vi "HEWH Solenoid Bank.vi"(0 "Test Fixture Hardware":T1={"Power "={"Yokogawa"={"WT210"={"Sample Rate (1: 0.25s)"=1, "A Range (12: 20A)"=11, "V Range (6: 600V)"=4, "Power VISA Yokogawa WT210"="WT210"}, "WT500"={"Power VISA Yokogawa WT500"="", "V Range (8: 1000V)"=6, "I Range (7: 40A)"=7, "Update Rate (3: 500ms)"=2}, "WT310_2"={"Sample Rate (1: 0.25s)"=1, "A Range (12: 20A)"=11, "V Range (6: 600V)"=4, "Power VISA Yokogawa WT310_2"="WT310_2"}, "WT310_3"={"Sample Rate (1: 0.25s)"=1, "A Range (12: 20A)"=11, "V Range (6: 600V)"=4, "Power VISA Yokogawa WT310_3"="WT310_3"}}, "Aplus"={"Aplus IP Address"="192.168.1.101", "Remote Port"=502, "Instrument"="APLUS", "Instr Driver Revision"="1.03.0053"}, "Power Limits"={"Crest Factor"={"Upper Limit"=1.49, "Lower Limit"=1.34}, "Harmonic Content"={"Uthd"=2.0}, "Voltage"={"% Error"=2.0}, "Stability"={"<1 Watt "={"Wattage"=1.0, "Slope (mW/H)"=10.0}, ">1 Watt"={"1%Power/Hour"=1.0}}}, "Nominal Voltage"=120, "Time Limit (s)"=10800.0, "Power Variation Limit (%)"=50.0, "Power Supply"={"Chroma 61605"="CHROMA", "Use Chroma?"=FALSE}}, "Weight Scale"={"Com Options"={"IND560Scale VISA"="IND560", "IP Address"="", "Remote Port"=502, "Setra Scale VISA"="SETRA", "GSE 350"="GSE350"}, "Select Scale"=""}, "Flow Rates"={"Laurel Cold IP Address"="", "Laurel Hot IP Address"="", "Hot Water Laurel VISA"="LaurelMeter_Hot", "Cold Water Laurel VISA"="LaurelMeter_Cold", "Remote Port"=0, "Laurel Communication Type"="", "Meters To Collect (Hot Cold)"="", "HOT Laurel Reference"=refnum, "COLD Laurel Reference"=refnum, "Modbus Hot Ref"=refnum}, "Analog Data"={"Agilent"={"Agilent 34972_1"="34972A_1", "Agilent 34972_2"="34972A_2", "Agilent 34972_3"="34972A_3", "Agilent 34972_4"="34972A_3", "Agilent 34972_5"="34972A_3", "Agilent 34972_6"="34972A_3", "Agilent Gain"=0.0, "TC Type (K,J,T)"="", "Instrument IDN?"="", "TC Channels-List"="", "Analog Channels-List"="", "Agilent Cluster Array"=[], "TC Channels-List 2"="", "Analog Channels-List 2"=""}, "Yokogawa"={"MW100"="MW100", "Intellifaucet"=FALSE}, "Select Analog"="", "TC Coefficients"={"TC Coefficients 1"=[], "TC Coefficients 2"=[], "TC Coefficients 3"=[], "TC Coefficients 4"=[], "TC Coefficients 5"=[], "TC Coefficients 6"=[], "TC Coefficients 7"=[]}, "NI Tasks (Dryer DOE)"=["TC Temps-Module 1", "TC Temps-Module 2", "TC Temps-Module 3", "TC Temps-Module 4", "TC Temps-Module 5", "Gas and Temp-Module 6", "AC_DC Events-Module 7"], "Laurel Analog"={"Laurel IP (Water Temp)"="", "Laurel IP (Pressure)"=""}}, "Viasala Temperature & Humidity"={"IP Address 1"="", "Remote Port"=0, "IP Address 2"="", "IP Address 3"="", "Viasala Modbus"=refnum, "Probe Number"=0}, "Gas Meter"={"Gas Meter 1"="COM3", "Gas Meter 2"="COM4", "Gas Meter 3"="COM5", "Gas Meter 4"="COM6", "Gas Meter 5"="COM7", "Gas Meter 6"="COM8", "Data Frame Format"={"Absolute Pressure"=FALSE, "Gauge/Diff. Pressure"=FALSE, "Barometric Pressure"=FALSE, "Temperature"=FALSE, "Volumetric"=FALSE, "Mass"=FALSE, "Setpoint"=FALSE, "Valve Drive"=FALSE, "Totalizer"=FALSE, "Totalizer Timer"=FALSE, "Totalizer Average Flow"=FALSE, "Totalizer Peak Flow"=FALSE, "Gas Selected"=FALSE, "Tot. Timer Format"=0}, "Measurement Units"={"Software Rev"="", "Model Number"="", "Manufacturer Info"="", "Software Sub-Rev"="", "Board Rev"="", "Units of Measure Input"={"Abs. Pressure"="", "Gauge/Diff. Press."="", "Barometric Press."="", "Temperature"="", "Volume"="", "Mass"="", "Setpoint"="", "Valve Drive"="", "Totalizer"="", "Tot. Timer"="", "Tot. Avg. Flow"="", "Tot. Peak Flow"=""}}, "Ritter Gas Meter 1"="COM8"}, "Barometric Pressure"={"HEISE 901A"="HEISE", "Use Barometer?"=FALSE}, "Gas Analysis"={"Ultramat 23 VISA"="ULTRAMAT"}, "Inficon Micro GC"={"Propane IP Address"="192.168.1.33", "Natural Gas  IP Address"="192.168.1.32", "Remote Port"=502, "Natural Modbus"=refnum, "Propane Modbus"=refnum}, "Tenney Environmental Chamber"={"Remote Port"=0, "IP Address"="", "Tenney Modbus"=refnum}} {"Power"."Yokogawa"."WT310_3"."V Range (6: 600V)" items=["Auto", "15V", "30V", "60V", "150V", "300V", "600V"]; "Power"."Yokogawa"."WT310_3"."A Range (12: 20A)" items=["Auto", "5mA", "10mA", "20mA", "50mA", "100mA", "200mA", "0.5A", "1A", "2A", "5A", "10A", "20A", "50mV", "100mV", "200mV", "2.5V", "5V", "10V"]; "Power"."Yokogawa"."WT310_3"."Sample Rate (1: 0.25s)" items=["0.1s", "0.25s", "0.5s", "1s", "2s", "5s"]; "Power"."Yokogawa"."WT310_2"."V Range (6: 600V)" items=["Auto", "15V", "30V", "60V", "150V", "300V", "600V"]; "Power"."Yokogawa"."WT310_2"."A Range (12: 20A)" items=["Auto", "5mA", "10mA", "20mA", "50mA", "100mA", "200mA", "0.5A", "1A", "2A", "5A", "10A", "20A", "50mV", "100mV", "200mV", "2.5V", "5V", "10V"]; "Power"."Yokogawa"."WT310_2"."Sample Rate (1: 0.25s)" items=["0.1s", "0.25s", "0.5s", "1s", "2s", "5s"]; "Power"."Yokogawa"."WT500"."Update Rate (3: 500ms)" items=["-", "100ms", "200ms", "500ms", "1s", "2s", "5s"]; "Power"."Yokogawa"."WT500"."I Range (7: 40A)" items=["AUTO", "500 mA", "1 A", "2 A", "5 A", "10 A", "20 A", "40 A", "S-AUTO", "50 mV", "100 mV", "200 mV", "500 mV", "1 V", "2 V", "5 V", "10 V", "250 mA", "500 mA", "1 A", "2.5 A", "5 A", "10 A", "20 A", "25 mV", "50 mV", "100 mV", "250 mV", "500 mV", "1 V", "2.5 V", "5 V"]; "Power"."Yokogawa"."WT500"."V Range (8: 1000V)" items=["AUTO", "15", "30", "60", "100", "150", "300", "600", "1000", "7.5", "15", "30", "50", "75", "150", "300", "500"]; "Power"."Yokogawa"."WT210"."V Range (6: 600V)" items=["Auto", "15V", "30V", "60V", "150V", "300V", "600V"]; "Power"."Yokogawa"."WT210"."A Range (12: 20A)" items=["Auto", "5mA", "10mA", "20mA", "50mA", "100mA", "200mA", "0.5A", "1A", "2A", "5A", "10A", "20A", "50mV", "100mV", "200mV", "2.5V", "5V", "10V"]; "Power"."Yokogawa"."WT210"."Sample Rate (1: 0.25s)" items=["0.1s", "0.25s", "0.5s", "1s", "2s", "5s"]}, 1 "Valve Bank Setting":T15, 2 "Station ID":T14=enum."A", 5 "Pressurize Tank while Heating?":bool, 11 "Error In":errorcluster, 12 "Debug":bool, 13 "Refnum in":T13, 14 "Disable Purge Pressurization":bool) -> (4 "Test Fixture Hardware Output":T1={"Power "={"Yokogawa"={"WT210"={"Sample Rate (1: 0.25s)"=1, "A Range (12: 20A)"=11, "V Range (6: 600V)"=4, "Power VISA Yokogawa WT210"="WT210"}, "WT500"={"Power VISA Yokogawa WT500"="", "V Range (8: 1000V)"=6, "I Range (7: 40A)"=7, "Update Rate (3: 500ms)"=2}, "WT310_2"={"Sample Rate (1: 0.25s)"=1, "A Range (12: 20A)"=11, "V Range (6: 600V)"=4, "Power VISA Yokogawa WT310_2"="WT310_2"}, "WT310_3"={"Sample Rate (1: 0.25s)"=1, "A Range (12: 20A)"=11, "V Range (6: 600V)"=4, "Power VISA Yokogawa WT310_3"="WT310_3"}}, "Aplus"={"Aplus IP Address"="192.168.1.101", "Remote Port"=502, "Instrument"="APLUS", "Instr Driver Revision"="1.03.0053"}, "Power Limits"={"Crest Factor"={"Upper Limit"=1.49, "Lower Limit"=1.34}, "Harmonic Content"={"Uthd"=2.0}, "Voltage"={"% Error"=2.0}, "Stability"={"<1 Watt "={"Wattage"=1.0, "Slope (mW/H)"=10.0}, ">1 Watt"={"1%Power/Hour"=1.0}}}, "Nominal Voltage"=120, "Time Limit (s)"=10800.0, "Power Variation Limit (%)"=50.0, "Power Supply"={"Chroma 61605"="CHROMA", "Use Chroma?"=FALSE}}, "Weight Scale"={"Com Options"={"IND560Scale VISA"="IND560", "IP Address"="", "Remote Port"=502, "Setra Scale VISA"="SETRA", "GSE 350"="GSE350"}, "Select Scale"=""}, "Flow Rates"={"Laurel Cold IP Address"="", "Laurel Hot IP Address"="", "Hot Water Laurel VISA"="LaurelMeter_Hot", "Cold Water Laurel VISA"="LaurelMeter_Cold", "Remote Port"=0, "Laurel Communication Type"="", "Meters To Collect (Hot Cold)"="", "HOT Laurel Reference"=refnum, "COLD Laurel Reference"=refnum, "Modbus Hot Ref"=refnum}, "Analog Data"={"Agilent"={"Agilent 34972_1"="34972A_1", "Agilent 34972_2"="34972A_2", "Agilent 34972_3"="34972A_3", "Agilent 34972_4"="34972A_3", "Agilent 34972_5"="34972A_3", "Agilent 34972_6"="34972A_3", "Agilent Gain"=0.0, "TC Type (K,J,T)"="", "Instrument IDN?"="", "TC Channels-List"="", "Analog Channels-List"="", "Agilent Cluster Array"=[], "TC Channels-List 2"="", "Analog Channels-List 2"=""}, "Yokogawa"={"MW100"="MW100", "Intellifaucet"=FALSE}, "Select Analog"="", "TC Coefficients"={"TC Coefficients 1"=[], "TC Coefficients 2"=[], "TC Coefficients 3"=[], "TC Coefficients 4"=[], "TC Coefficients 5"=[], "TC Coefficients 6"=[], "TC Coefficients 7"=[]}, "NI Tasks (Dryer DOE)"=["TC Temps-Module 1", "TC Temps-Module 2", "TC Temps-Module 3", "TC Temps-Module 4", "TC Temps-Module 5", "Gas and Temp-Module 6", "AC_DC Events-Module 7"], "Laurel Analog"={"Laurel IP (Water Temp)"="", "Laurel IP (Pressure)"=""}}, "Viasala Temperature & Humidity"={"IP Address 1"="", "Remote Port"=0, "IP Address 2"="", "IP Address 3"="", "Viasala Modbus"=refnum, "Probe Number"=0}, "Gas Meter"={"Gas Meter 1"="COM3", "Gas Meter 2"="COM4", "Gas Meter 3"="COM5", "Gas Meter 4"="COM6", "Gas Meter 5"="COM7", "Gas Meter 6"="COM8", "Data Frame Format"={"Absolute Pressure"=FALSE, "Gauge/Diff. Pressure"=FALSE, "Barometric Pressure"=FALSE, "Temperature"=FALSE, "Volumetric"=FALSE, "Mass"=FALSE, "Setpoint"=FALSE, "Valve Drive"=FALSE, "Totalizer"=FALSE, "Totalizer Timer"=FALSE, "Totalizer Average Flow"=FALSE, "Totalizer Peak Flow"=FALSE, "Gas Selected"=FALSE, "Tot. Timer Format"=0}, "Measurement Units"={"Software Rev"="", "Model Number"="", "Manufacturer Info"="", "Software Sub-Rev"="", "Board Rev"="", "Units of Measure Input"={"Abs. Pressure"="", "Gauge/Diff. Press."="", "Barometric Press."="", "Temperature"="", "Volume"="", "Mass"="", "Setpoint"="", "Valve Drive"="", "Totalizer"="", "Tot. Timer"="", "Tot. Avg. Flow"="", "Tot. Peak Flow"=""}}, "Ritter Gas Meter 1"="COM8"}, "Barometric Pressure"={"HEISE 901A"="HEISE", "Use Barometer?"=FALSE}, "Gas Analysis"={"Ultramat 23 VISA"="ULTRAMAT"}, "Inficon Micro GC"={"Propane IP Address"="192.168.1.33", "Natural Gas  IP Address"="192.168.1.32", "Remote Port"=502, "Natural Modbus"=refnum, "Propane Modbus"=refnum}, "Tenney Environmental Chamber"={"Remote Port"=0, "IP Address"="", "Tenney Modbus"=refnum}} {"Power"."Yokogawa"."WT310_3"."V Range (6: 600V)" items=["Auto", "15V", "30V", "60V", "150V", "300V", "600V"]; "Power"."Yokogawa"."WT310_3"."A Range (12: 20A)" items=["Auto", "5mA", "10mA", "20mA", "50mA", "100mA", "200mA", "0.5A", "1A", "2A", "5A", "10A", "20A", "50mV", "100mV", "200mV", "2.5V", "5V", "10V"]; "Power"."Yokogawa"."WT310_3"."Sample Rate (1: 0.25s)" items=["0.1s", "0.25s", "0.5s", "1s", "2s", "5s"]; "Power"."Yokogawa"."WT310_2"."V Range (6: 600V)" items=["Auto", "15V", "30V", "60V", "150V", "300V", "600V"]; "Power"."Yokogawa"."WT310_2"."A Range (12: 20A)" items=["Auto", "5mA", "10mA", "20mA", "50mA", "100mA", "200mA", "0.5A", "1A", "2A", "5A", "10A", "20A", "50mV", "100mV", "200mV", "2.5V", "5V", "10V"]; "Power"."Yokogawa"."WT310_2"."Sample Rate (1: 0.25s)" items=["0.1s", "0.25s", "0.5s", "1s", "2s", "5s"]; "Power"."Yokogawa"."WT500"."Update Rate (3: 500ms)" items=["-", "100ms", "200ms", "500ms", "1s", "2s", "5s"]; "Power"."Yokogawa"."WT500"."I Range (7: 40A)" items=["AUTO", "500 mA", "1 A", "2 A", "5 A", "10 A", "20 A", "40 A", "S-AUTO", "50 mV", "100 mV", "200 mV", "500 mV", "1 V", "2 V", "5 V", "10 V", "250 mA", "500 mA", "1 A", "2.5 A", "5 A", "10 A", "20 A", "25 mV", "50 mV", "100 mV", "250 mV", "500 mV", "1 V", "2.5 V", "5 V"]; "Power"."Yokogawa"."WT500"."V Range (8: 1000V)" items=["AUTO", "15", "30", "60", "100", "150", "300", "600", "1000", "7.5", "15", "30", "50", "75", "150", "300", "500"]; "Power"."Yokogawa"."WT210"."V Range (6: 600V)" items=["Auto", "15V", "30V", "60V", "150V", "300V", "600V"]; "Power"."Yokogawa"."WT210"."A Range (12: 20A)" items=["Auto", "5mA", "10mA", "20mA", "50mA", "100mA", "200mA", "0.5A", "1A", "2A", "5A", "10A", "20A", "50mV", "100mV", "200mV", "2.5V", "5V", "10V"]; "Power"."Yokogawa"."WT210"."Sample Rate (1: 0.25s)" items=["0.1s", "0.25s", "0.5s", "1s", "2s", "5s"]}, 6 "Input Valve Output":T12="ON", 8 "Drain/Purge Valve Output":T11="OFF", 10 "Outlet Valve Output":T12="OFF", 15 "Error Out":errorcluster)   [LabVIEW 2023]
uses:
  Type Definitions/HEWH MW100 Channel Numbers.ctl
  Type Definitions/HEWH Valve Bank Positions.ctl
  Type Definitions/Station ID Selector.ctl
  Type Definitions/HEWH Normally Open Valve Control.ctl
  Type Definitions/HEWH Normally Closed Valve Control.ctl
  Utility/Type Definitions/UTILITY Power Inputs Control.ctl
  Drivers/IND560 Scale Monitor/Type Definitions/IND560 Configuration.ctl
  Type Definitions/HEWH Agilent Cluster.ctl
  Utility/Type Definitions/UTILITY TC Coefficients.ctl
  Drivers/Alicat Gas Meter Driver/Sub-VIs/Data Frame.ctl
  Drivers/Alicat Gas Meter Driver/Sub-VIs/Units of Measure.ctl
  Drivers/Omega FMA-1600A Series Gas Flow Meter/Type Definitions/FMA1600A Units String.ctl
  Drivers/Omega FMA-1600A Series Gas Flow Meter/Type Definitions/FMA1600A COM Ports.ctl
  Washer DOE/Type Definitions/DOE Test Fixture Hardware.ctl
  <vilib>/NI/Modbus Library/API/Master/Modbus Master.lvclass
  Drivers/Inficon Fusion Micro GC/Type Definitions/Inficon IP Address.ctl
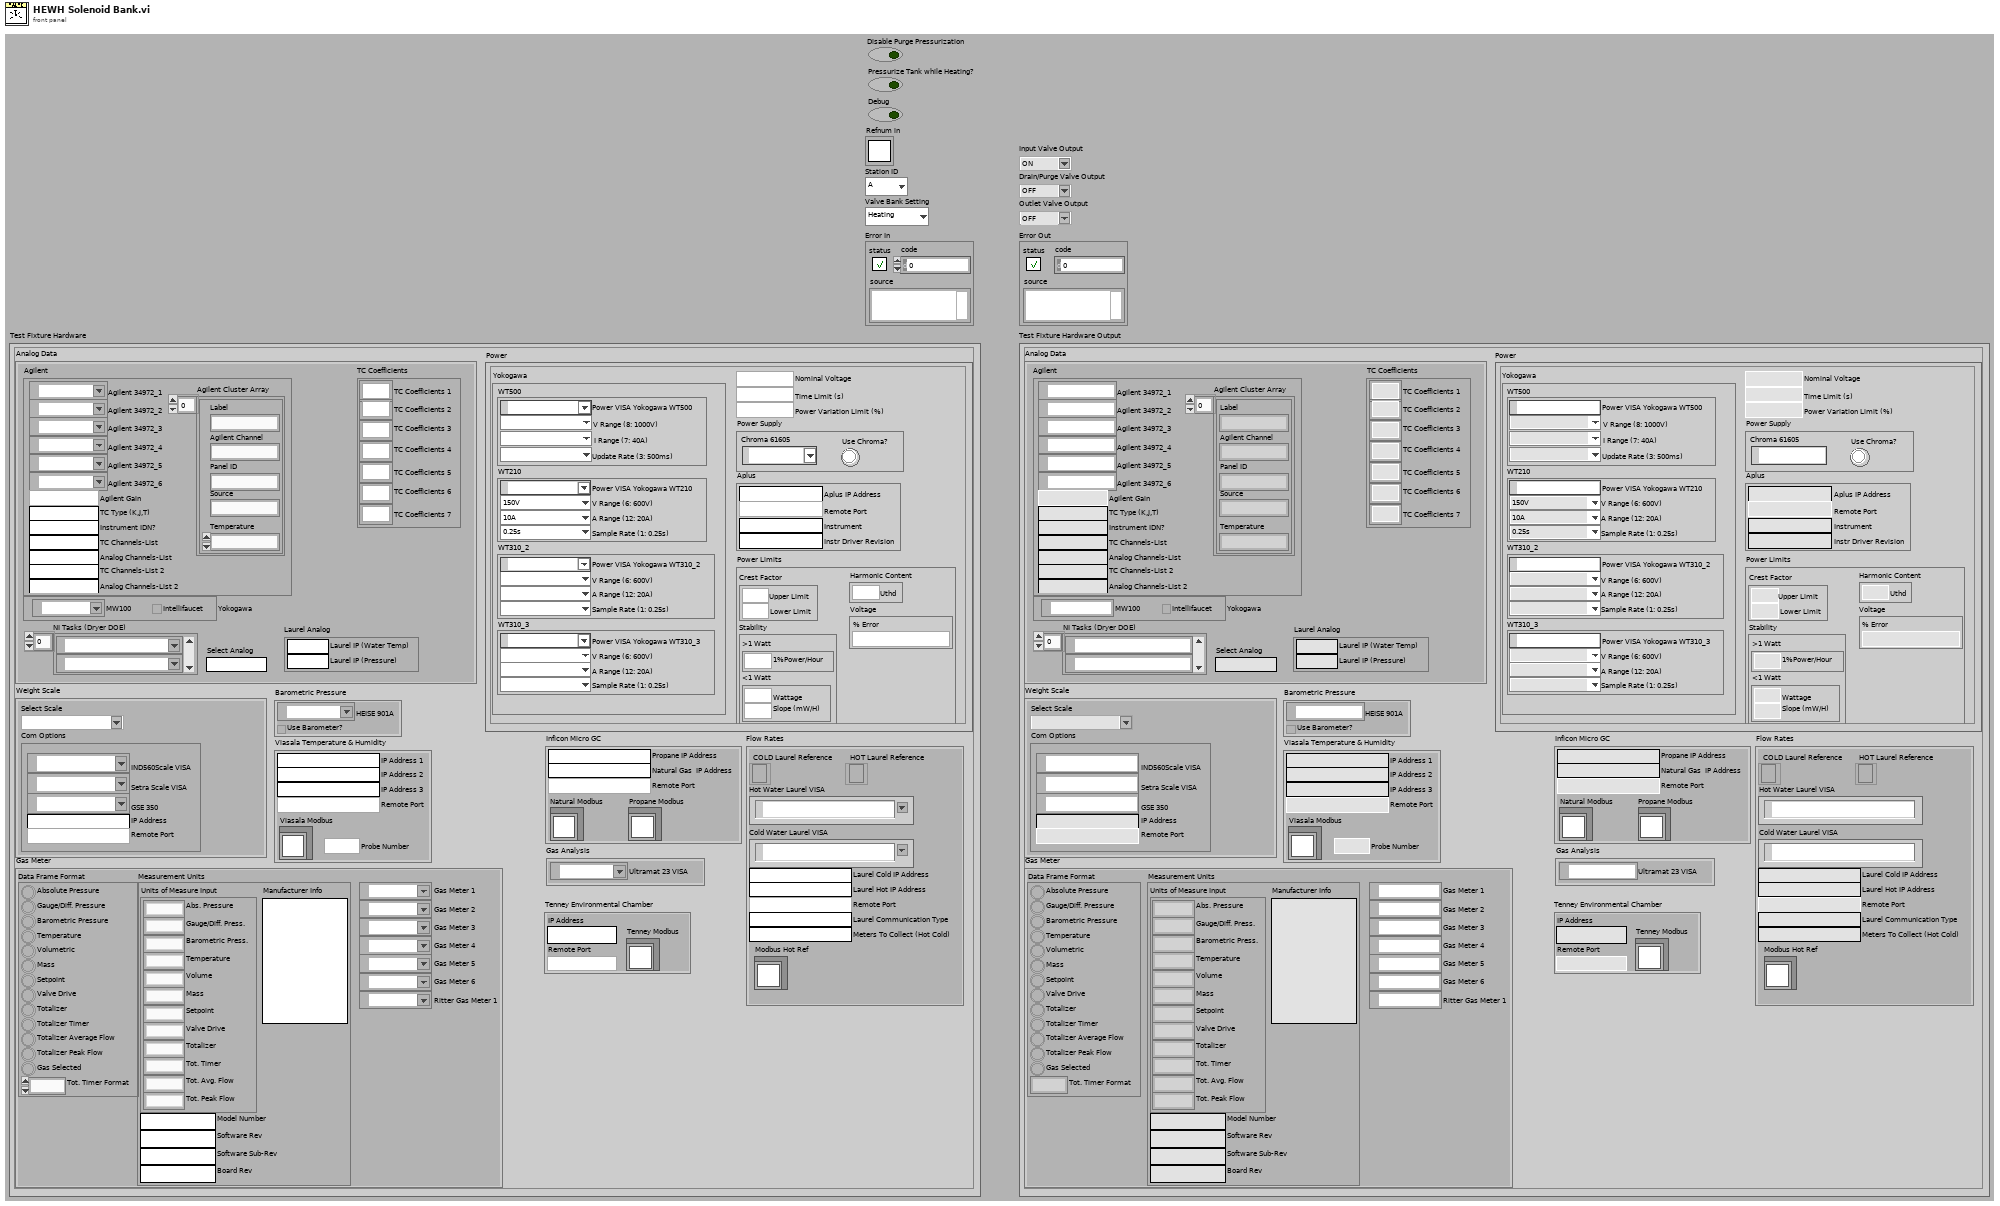
[diagram p1: front panel]
types:
  T1 = typedef "DOE Test Fixture Hardware.ctl" = cluster{"Power ":T2, "Weight Scale":cluster{"Com Options":T3, "Select Scale":string}, "Flow Rates":cluster{"Laurel Cold IP Address":string, "Laurel Hot IP Address":string, "Hot Water Laurel VISA":refnum<visa-resource-name>, "Cold Water Laurel VISA":refnum<visa-resource-name>, "Remote Port":u16, "Laurel Communication Type":string, "Meters To Collect (Hot Cold)":string, "HOT Laurel Reference":refnum<k5>, "COLD Laurel Reference":refnum<k5>, "Modbus Hot Ref":refnum<class "Modbus Master.lvclass">}, "Analog Data":cluster{"Agilent":cluster{"Agilent 34972_1":refnum<visa-resource-name>, "Agilent 34972_2":refnum<visa-resource-name>, "Agilent 34972_3":refnum<visa-resource-name>, "Agilent 34972_4":refnum<visa-resource-name>, "Agilent 34972_5":refnum<visa-resource-name>, "Agilent 34972_6":refnum<visa-resource-name>, "Agilent Gain":dbl, "TC Type (K,J,T)":string, "Instrument IDN?":string, "TC Channels-List":string, "Analog Channels-List":string, "Agilent Cluster Array":T4[], "TC Channels-List 2":string, "Analog Channels-List 2":string}, "Yokogawa":cluster{"MW100":refnum<visa-resource-name>, "Intellifaucet":bool}, "Select Analog":string, "TC Coefficients":T5, "NI Tasks (Dryer DOE)":refnum<k21>[], "Laurel Analog":cluster{"Laurel IP (Water Temp)":string, "Laurel IP (Pressure)":string}}, "Viasala Temperature & Humidity":cluster{"IP Address 1":string, "Remote Port":u16, "IP Address 2":string, "IP Address 3":string, "Viasala Modbus":refnum<class "Modbus Master.lvclass">, "Probe Number":u16}, "Gas Meter":T6, "Barometric Pressure":cluster{"HEISE 901A":refnum<visa-resource-name>, "Use Barometer?":bool}, "Gas Analysis":cluster{"Ultramat 23 VISA":refnum<visa-resource-name>}, "Inficon Micro GC":T10, "Tenney Environmental Chamber":cluster{"Remote Port":u16, "IP Address":string, "Tenney Modbus":refnum<class "Modbus Master.lvclass">}}
  T2 = typedef "UTILITY Power Inputs Control.ctl" = cluster{"Yokogawa":cluster{"WT210":cluster{"Sample Rate (1: 0.25s)":i32, "A Range (12: 20A)":i32, "V Range (6: 600V)":i32, "Power VISA Yokogawa WT210":refnum<visa-resource-name>}, "WT500":cluster{"Power VISA Yokogawa WT500":refnum<visa-resource-name>, "V Range (8: 1000V)":i32, "I Range (7: 40A)":i32, "Update Rate (3: 500ms)":i32}, "WT310_2":cluster{"Sample Rate (1: 0.25s)":i32, "A Range (12: 20A)":i32, "V Range (6: 600V)":i32, "Power VISA Yokogawa WT310_2":refnum<visa-resource-name>}, "WT310_3":cluster{"Sample Rate (1: 0.25s)":i32, "A Range (12: 20A)":i32, "V Range (6: 600V)":i32, "Power VISA Yokogawa WT310_3":refnum<visa-resource-name>}}, "Aplus":cluster{"Aplus IP Address":string, "Remote Port":i32, "Instrument":string, "Instr Driver Revision":string}, "Power Limits":cluster{"Crest Factor":cluster{"Upper Limit":dbl, "Lower Limit":dbl}, "Harmonic Content":cluster{"Uthd":dbl}, "Voltage":cluster{"% Error":dbl}, "Stability":cluster{"<1 Watt ":cluster{"Wattage":dbl, "Slope (mW/H)":dbl}, ">1 Watt":cluster{"1%Power/Hour":dbl}}}, "Nominal Voltage":i32, "Time Limit (s)":dbl, "Power Variation Limit (%)":dbl, "Power Supply":cluster{"Chroma 61605":refnum<visa-resource-name>, "Use Chroma?":bool}}
  T3 = typedef "IND560 Configuration.ctl" = cluster{"IND560Scale VISA":refnum<visa-resource-name>, "IP Address":string, "Remote Port":u16, "Setra Scale VISA":refnum<visa-resource-name>, "GSE 350":refnum<visa-resource-name>}
  T4 = typedef "HEWH Agilent Cluster.ctl" = cluster{"Label":string, "Agilent Channel":string, "Panel ID":string, "Source":string, "Temperature":dbl}
  T5 = typedef "UTILITY TC Coefficients.ctl" = cluster{"TC Coefficients 1":dbl[], "TC Coefficients 2":dbl[], "TC Coefficients 3":dbl[], "TC Coefficients 4":dbl[], "TC Coefficients 5":dbl[], "TC Coefficients 6":dbl[], "TC Coefficients 7":dbl[]}
  T6 = typedef "FMA1600A COM Ports.ctl" = cluster{"Gas Meter 1":refnum<visa-resource-name>, "Gas Meter 2":refnum<visa-resource-name>, "Gas Meter 3":refnum<visa-resource-name>, "Gas Meter 4":refnum<visa-resource-name>, "Gas Meter 5":refnum<visa-resource-name>, "Gas Meter 6":refnum<visa-resource-name>, "Data Frame Format":T7, "Measurement Units":T8, "Ritter Gas Meter 1":refnum<visa-resource-name>}
  T7 = typedef "Data Frame.ctl" = cluster{"Absolute Pressure":bool, "Gauge/Diff. Pressure":bool, "Barometric Pressure":bool, "Temperature":bool, "Volumetric":bool, "Mass":bool, "Setpoint":bool, "Valve Drive":bool, "Totalizer":bool, "Totalizer Timer":bool, "Totalizer Average Flow":bool, "Totalizer Peak Flow":bool, "Gas Selected":bool, "Tot. Timer Format":u16}
  T8 = typedef "FMA1600A Units String.ctl" = cluster{"Software Rev":string, "Model Number":string, "Manufacturer Info":string, "Software Sub-Rev":string, "Board Rev":string, "Units of Measure Input":T9}
  T9 = typedef "Units of Measure.ctl" = cluster{"Abs. Pressure":string, "Gauge/Diff. Press.":string, "Barometric Press.":string, "Temperature":string, "Volume":string, "Mass":string, "Setpoint":string, "Valve Drive":string, "Totalizer":string, "Tot. Timer":string, "Tot. Avg. Flow":string, "Tot. Peak Flow":string}
  T10 = typedef "Inficon IP Address.ctl" = cluster{"Propane IP Address":string, "Natural Gas  IP Address":string, "Remote Port":u16, "Natural Modbus":refnum<class "Modbus Master.lvclass">, "Propane Modbus":refnum<class "Modbus Master.lvclass">}
  T11 = typedef "HEWH Normally Closed Valve Control.ctl" = string
  T12 = typedef "HEWH Normally Open Valve Control.ctl" = string
  T13 = typedef "Semaphore RefNum" = refnum<k1>
  T14 = typedef "Station ID Selector.ctl" = enum16{"", "A", "B", "C", "D", "Global"}
  T15 = typedef "HEWH Valve Bank Positions.ctl" = enum16{"Heating", "Purge", "Resting", "Draw"}
  T16 = typedef "HEWH MW100 Channel Numbers.ctl" = string
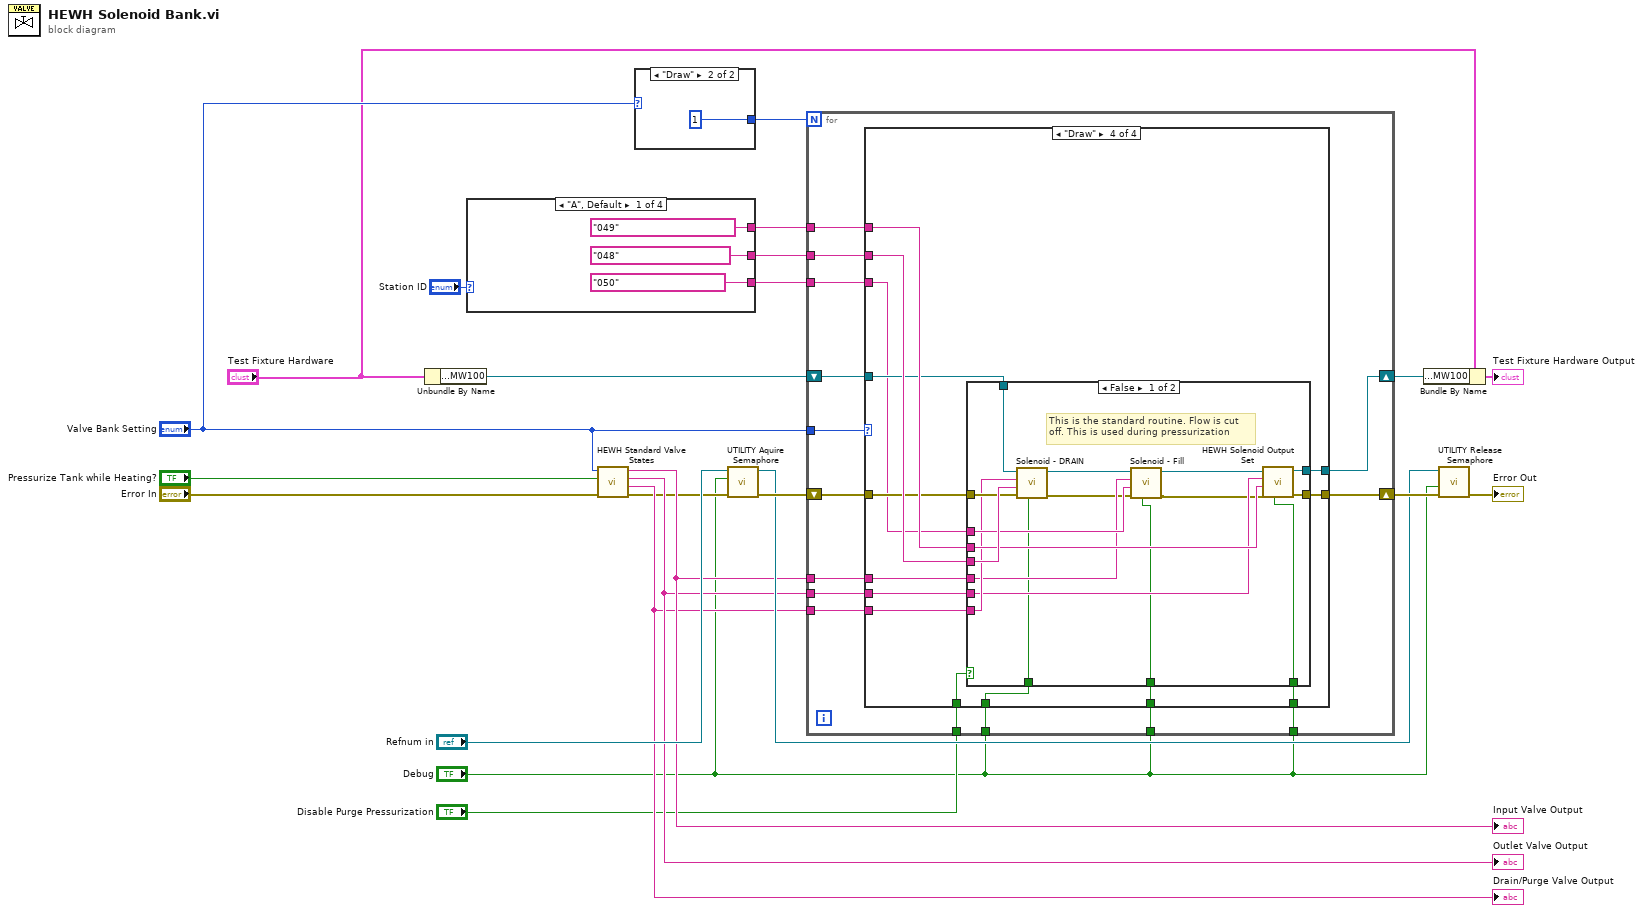
[diagram p0: block diagram]
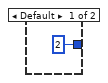
[diagram p2: hidden frame]
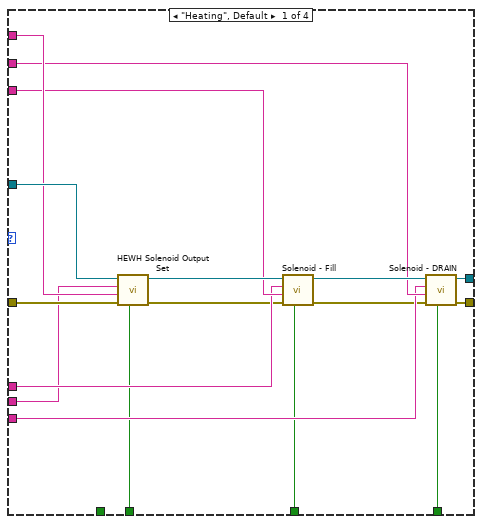
[diagram p3: hidden frame]
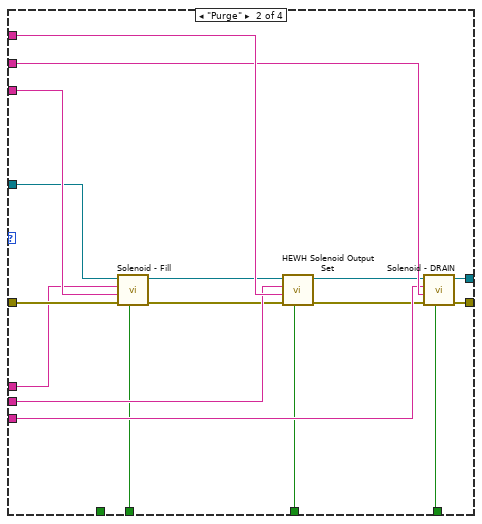
[diagram p4: hidden frame]
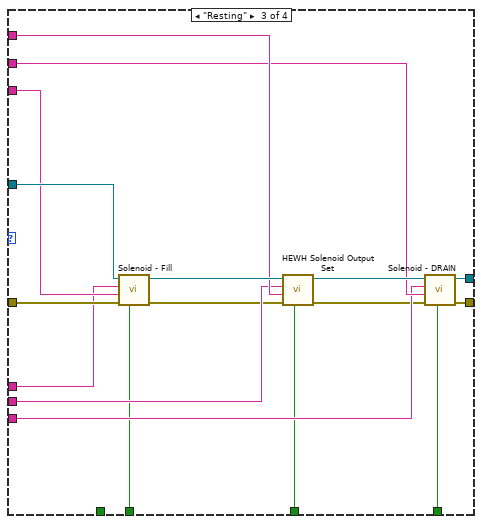
[diagram p5: hidden frame]
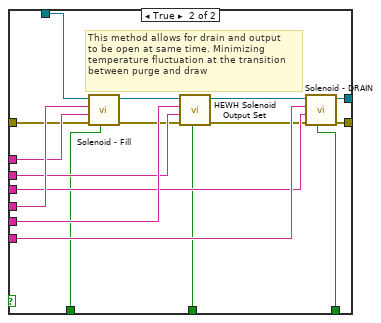
[diagram p6: hidden frame]
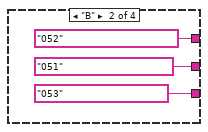
[diagram p7: hidden frame]
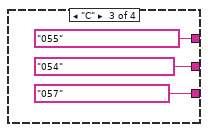
[diagram p8: hidden frame]
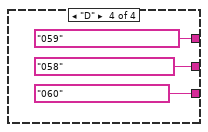
[diagram p9: hidden frame]
diagram:
  n1 = Unbundle By Name("Test Fixture Hardware") -> ("Analog Data.Yokogawa.MW100"=w6:refnum<visa-resource-name>)
  n2 = case shown="\"A\", Default" "Station ID" {
    tunnel: [T16 "048" ("HEWH MW100 Channel Numbers") T16 "051" ("HEWH MW100 Channel Numbers") T16 "054" ("HEWH MW100 Channel Numbers") T16 "058" ("HEWH MW100 Channel Numbers")] -> w21
    tunnel: [T16 "049" ("HEWH MW100 Channel Numbers") T16 "052" ("HEWH MW100 Channel Numbers") T16 "055" ("HEWH MW100 Channel Numbers") T16 "059" ("HEWH MW100 Channel Numbers")] -> w23
    tunnel: [T16 "050" ("HEWH MW100 Channel Numbers") T16 "053" ("HEWH MW100 Channel Numbers") T16 "057" ("HEWH MW100 Channel Numbers") T16 "060" ("HEWH MW100 Channel Numbers")] -> w22
    frame "A", Default {
    }
    frame "B" {
    }
    frame "C" {
    }
    frame "D" {
    }
  }
  n3 = call "HEWH Standard Valve States.vi"("Error In"="Error In", "Pressurize Tank while Heating?"="Pressurize Tank while Heating?", "Valve Bank Setting"="Valve Bank Setting") -> ("Error Out"=w9:errorcluster, "Drain/Purge Valve"=w11:T11, "Outlet Valve"=w12:T12, "Input Valve"=w13:T12)  [unwired: 5 in]
  "Input Valve Output" <- w13
  "Outlet Valve Output" <- w12
  "Drain/Purge Valve Output" <- w11
  n4 = case shown="\"Draw\"" "Valve Bank Setting" {
    tunnel: [2 1] -> w8
    frame Default {
    }
    frame "Draw" {
    }
  }
  n5 = call "UTILITY Aquire Semaphore.vi"("error in (no error)"=w9, "Debug"="Debug", "Refnum in"="Refnum in") -> ("error out"=w17:errorcluster, "Refnum out"=w16:T13)  [unwired: 7 in]
  n6 = for {
    N: w8 -> [_]
    tunnel: w23 -> [w52]
    tunnel: w22 -> [w51]
    tunnel: w21 -> [w50]
    tunnel: "Valve Bank Setting" -> [w45]
    tunnel: w13 -> [w44]
    tunnel: w12 -> [w43]
    tunnel: w11 -> [w42]
    shift-right: [w49] -> w4
    shift-left: w6 -> [w48]
    shift-right: [w47] -> w19
    shift-left: w17 -> [w46]
    tunnel: "Disable Purge Pressurization" -> [w41]
    tunnel: "Debug" -> [w40]
    tunnel: "Debug" -> [w39]
    tunnel: "Debug" -> [w38]
    n7 = case shown="\"Draw\"" w45 {
      tunnel: w52 -> [w64 w86 w96 w116]
      tunnel: w51 -> [w63 w85 w97 w107]
      tunnel: w50 -> [w62 w84 w95 w117]
      tunnel: [w61 w81 w99 w109] -> w49
      tunnel: [w69 w80 w98 w110] -> w47
      tunnel: w46 -> [w68 w79 w103 w115]
      tunnel: w48 -> [w67 w78 w102 w114]
      tunnel: w44 -> [w60 w77 w94 w112]
      tunnel: w43 -> [w59 w76 w93 w111]
      tunnel: w42 -> [w58 w75 w92 w113]
      tunnel: w41 -> [_ _ _ w108]
      tunnel: w40 -> [w55 w72 w89 w106]
      tunnel: w39 -> [w54 w71 w88 w105]
      tunnel: w38 -> [w53 w70 w87 w104]
      frame "Heating", Default {
        n8 = call "HEWH Solenoid Output Set.vi"("Debug"=w55, "Error In"=w68, "HEWH MW100 Channel Numbers"=w64, "Outlet Valve"=w59, "VISA session"=w67) -> ("Error Out"=w57:errorcluster, "dup VISA session"=w66:refnum<visa-resource-name>)  [unwired: 5 in]
        n9 = call "Solenoid - Fill.vi"("Debug"=w54, "Error In"=w57, "HEWH MW100 Channel Numbers"=w63, "Input Valve"=w60, "VISA session"=w66) -> ("Error Out"=w56:errorcluster, "dup VISA session"=w65:refnum<visa-resource-name>)  [unwired: 5 in]
        n10 = call "Solenoid - DRAIN.vi"("Debug"=w53, "Error In"=w56, "HEWH MW100 Channel Numbers"=w62, "Drain/Purge Valve"=w58, "VISA session"=w65) -> ("Error Out"=w69:errorcluster, "dup VISA session"=w61:refnum<visa-resource-name>)  [unwired: 5 in]
      }
      frame "Purge" {
        n11 = call "Solenoid - Fill.vi"("Debug"=w72, "Error In"=w79, "HEWH MW100 Channel Numbers"=w85, "Input Valve"=w77, "VISA session"=w78) -> ("Error Out"=w74:errorcluster, "dup VISA session"=w82:refnum<visa-resource-name>)  [unwired: 5 in]
        n12 = call "HEWH Solenoid Output Set.vi"("Debug"=w71, "Error In"=w74, "HEWH MW100 Channel Numbers"=w86, "Outlet Valve"=w76, "VISA session"=w82) -> ("Error Out"=w73:errorcluster, "dup VISA session"=w83:refnum<visa-resource-name>)  [unwired: 5 in]
        n13 = call "Solenoid - DRAIN.vi"("Debug"=w70, "Error In"=w73, "HEWH MW100 Channel Numbers"=w84, "Drain/Purge Valve"=w75, "VISA session"=w83) -> ("Error Out"=w80:errorcluster, "dup VISA session"=w81:refnum<visa-resource-name>)  [unwired: 5 in]
      }
      frame "Resting" {
        n14 = call "Solenoid - Fill.vi"("Debug"=w89, "Error In"=w103, "HEWH MW100 Channel Numbers"=w97, "Input Valve"=w94, "VISA session"=w102) -> ("Error Out"=w91:errorcluster, "dup VISA session"=w101:refnum<visa-resource-name>)  [unwired: 5 in]
        n15 = call "HEWH Solenoid Output Set.vi"("Debug"=w88, "Error In"=w91, "HEWH MW100 Channel Numbers"=w96, "Outlet Valve"=w93, "VISA session"=w101) -> ("Error Out"=w90:errorcluster, "dup VISA session"=w100:refnum<visa-resource-name>)  [unwired: 5 in]
        n16 = call "Solenoid - DRAIN.vi"("Debug"=w87, "Error In"=w90, "HEWH MW100 Channel Numbers"=w95, "Drain/Purge Valve"=w92, "VISA session"=w100) -> ("Error Out"=w98:errorcluster, "dup VISA session"=w99:refnum<visa-resource-name>)  [unwired: 5 in]
      }
      frame "Draw" {
        n17 = case shown="False" w108 {
          tunnel: w117 -> [w134 w148]
          tunnel: w116 -> [w133 w146]
          tunnel: w107 -> [w132 w147]
          tunnel: w115 -> [w131 w143]
          tunnel: w114 -> [w130 w142]
          tunnel: w113 -> [w129 w149]
          tunnel: w112 -> [w128 w151]
          tunnel: w111 -> [w127 w150]
          tunnel: [w126 w145] -> w110
          tunnel: [w125 w144] -> w109
          tunnel: w106 -> [w120 w137]
          tunnel: w105 -> [w119 w136]
          tunnel: w104 -> [w118 w135]
          frame False {
            # "This is the standard routine. Flow is cut\noff. This is used during pressurization"
            n18 = call "Solenoid - DRAIN.vi"("Debug"=w120, "Error In"=w131, "HEWH MW100 Channel Numbers"=w134, "Drain/Purge Valve"=w129, "VISA session"=w130) -> ("Error Out"=w122:errorcluster, "dup VISA session"=w123:refnum<visa-resource-name>)  [unwired: 5 in]
            n19 = call "Solenoid - Fill.vi"("Debug"=w119, "Error In"=w122, "HEWH MW100 Channel Numbers"=w132, "Input Valve"=w128, "VISA session"=w123) -> ("Error Out"=w121:errorcluster, "dup VISA session"=w124:refnum<visa-resource-name>)  [unwired: 5 in]
            n20 = call "HEWH Solenoid Output Set.vi"("Debug"=w118, "Error In"=w121, "HEWH MW100 Channel Numbers"=w133, "Outlet Valve"=w127, "VISA session"=w124) -> ("Error Out"=w126:errorcluster, "dup VISA session"=w125:refnum<visa-resource-name>)  [unwired: 5 in]
          }
          frame True {
            # "This method allows for drain and output\nto be open at same time. Minimizing\ntemperature fluctuation at the transition\nbetween purge and draw"
            n21 = call "Solenoid - Fill.vi"("Debug"=w137, "Error In"=w143, "HEWH MW100 Channel Numbers"=w147, "Input Valve"=w151, "VISA session"=w142) -> ("Error Out"=w139:errorcluster, "dup VISA session"=w140:refnum<visa-resource-name>)  [unwired: 5 in]
            n22 = call "HEWH Solenoid Output Set.vi"("Debug"=w136, "Error In"=w139, "HEWH MW100 Channel Numbers"=w146, "Outlet Valve"=w150, "VISA session"=w140) -> ("Error Out"=w138:errorcluster, "dup VISA session"=w141:refnum<visa-resource-name>)  [unwired: 5 in]
            n23 = call "Solenoid - DRAIN.vi"("Debug"=w135, "Error In"=w138, "HEWH MW100 Channel Numbers"=w148, "Drain/Purge Valve"=w149, "VISA session"=w141) -> ("Error Out"=w145:errorcluster, "dup VISA session"=w144:refnum<visa-resource-name>)  [unwired: 5 in]
          }
        }
      }
    }
  }
  n24 = Bundle By Name(cluster="Test Fixture Hardware", "Analog Data.Yokogawa.MW100"=w4) -> (→"Test Fixture Hardware Output":T1)
  n25 = call "UTILITY Release Semaphore.vi"("error in (no error)"=w19, "Debug"="Debug", "Refnum in"=w16) -> ("error out"=→"Error Out":errorcluster)  [unwired: 8 in]
